vi "Configure Limit.vi"(7 "Enable Limit (F: Disable)":bool, 8 "error in (no error)":errorcluster, 9 "Upper Limit (0)":dbl, 10 "Lower Limit (0)":dbl, 11 "VISA resource name":refnum<visa-resource-name>) -> (0 "error out":errorcluster, 3 "VISA resource name out":refnum<visa-resource-name>)   [LabVIEW 2013, in "Agilent 3446X Series.lvlib"]
doc: "Configures the settings of limit testing."
uses:
  Agilent 3446X Series.lvlib
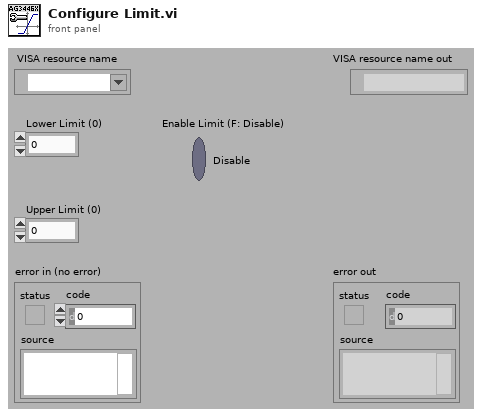
[diagram p1: front panel]
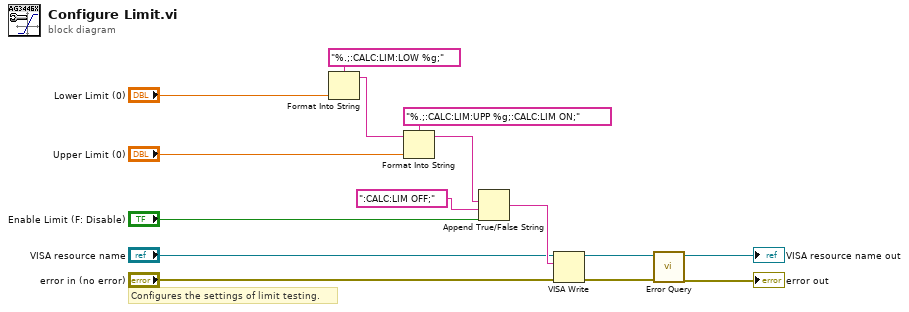
[diagram p0: block diagram]
diagram:
  # "Configures the settings of limit testing."
  n1 = Format Into String(format string="%.;:CALC:LIM:LOW %g;", "Lower Limit (0)") -> (resulting string=w13:string)  [unwired: 2 in, 1 out]
  n2 = Format Into String(format string="%.;:CALC:LIM:UPP %g;:CALC:LIM ON;", initial string=w13, "Upper Limit (0)") -> (resulting string=w1:string)  [unwired: 1 in, 1 out]
  n3 = Append True/False String(1:"Enable Limit (F: Disable)", 2:":CALC:LIM OFF;", 3:w1) -> (0:w8:string)  [unwired: 1 out]
  n4 = VISA Write(VISA resource name="VISA resource name", write buffer=w8, error in (no error)="error in (no error)") -> (VISA resource name out=w5:refnum<visa-resource-name>, error out=w4:errorcluster)  [unwired: 1 out]
  n5 = call "Error Query.vi"("error in (no error)"=w4, "VISA resource name"=w5) -> ("error out"=→"error out":errorcluster, "VISA resource name out"=→"VISA resource name out":refnum<visa-resource-name>)  [unwired: 8 out]
